vi "MB Embedded Modbus Demo Box Example.vi"() -> ()   [LabVIEW 2011]
uses:
  MB Serial Master Query Read Coils (poly).vi
  MB Serial Master Query Write Multiple Coils (poly).vi
  MB Serial Master Query Read Holding Registers (poly).vi
  MB Serial Master Query Write Multiple Registers (poly).vi
panel:
  in  "Stop":bool
  in  "COM Port":refnum<visa-resource-name>
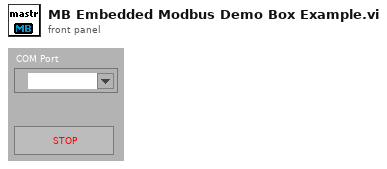
[diagram p1: front panel]
types:
  T1 = cluster{"Mode":enum16{"RTU", "ASCII"}, "Slave Address":u8}
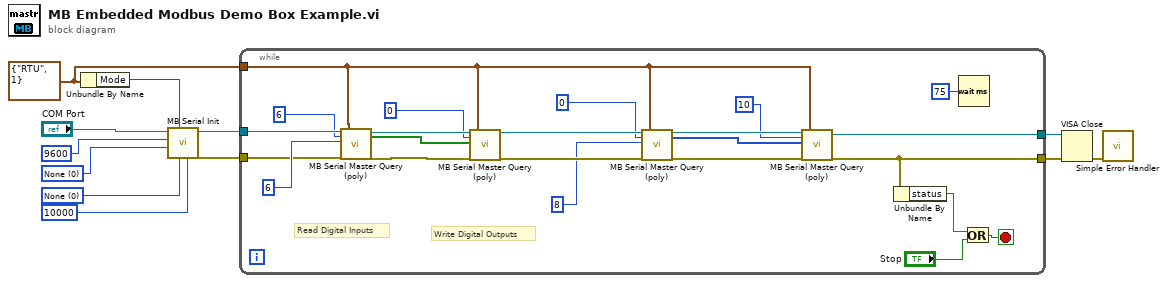
[diagram p0: block diagram]
diagram:
  w7 = u16 0 items=["None", "XON/XOFF", "RTS/CTS", "XON/XOFF & RTS/CTS", "DTR/DSR", "XON/XOFF & DTR/DSR"] ("Flow Control")
  w8 = u16 0 items=["None", "Odd", "Even", "Mark", "Space"] ("Parity")
  w4 = T1 {"Mode"=enum."RTU", "Slave Address"=1} ("Serial Parameters")
  n1 = Unbundle By Name(w4) -> ("Mode"=w10:enum16{"RTU", "ASCII"})
  n2 = call "MB Serial Init.vi"("Timeout"=u32 10000, "Flow Control"=w7, "Mode"=w10, "Parity"=w8, "Baud Rate"=u32 9600, "VISA resource name"="COM Port") -> ("error out"=w5:errorcluster, "VISA resource name out"=w11:refnum<visa-resource-name>)  [unwired: 1 in, 3 out]
  n3 = while {
    tunnel: w11 -> [w35]
    tunnel: w5 -> [w32]
    tunnel: w4 -> [w19]
    tunnel: [w15] -> w3
    tunnel: [w14] -> w2
    stop <- w18 stop-if-true
    # "Write Digital Outputs"
    # "Read Digital Inputs"
    n4 = call-poly "MB Serial Master Query (poly).vi"("VISA resource name"=w35, "Starting Address"=u16 6, "Quantity"=u16 6, "error in"=w32, "Serial Parameters"=w19) -> ("VISA resource name out"=w31:refnum<visa-resource-name>, "Coils"=w28:bool[], "error out"=w30:errorcluster)  [unwired: 1 in, 11 out]
    n5 = call-poly "MB Serial Master Query (poly).vi"("VISA resource name"=w31, "Starting Address"=u16 0, "Coils"=w28, "error in"=w30, "Serial Parameters"=w19) -> ("VISA resource name out"=w27:refnum<visa-resource-name>, "error out"=w26:errorcluster)  [unwired: 2 in, 11 out]
    n6 = call-poly "MB Serial Master Query (poly).vi"("VISA resource name"=w27, "Starting Address"=u16 0, "Quantity"=u16 8, "error in"=w26, "Serial Parameters"=w19) -> ("VISA resource name out"=w23:refnum<visa-resource-name>, "Holding Registers"=w20:u16[], "error out"=w22:errorcluster)  [unwired: 1 in, 11 out]
    n7 = call-poly "MB Serial Master Query (poly).vi"("VISA resource name"=w23, "Starting Address"=u16 10, "Registers"=w20, "error in"=w22, "Serial Parameters"=w19) -> ("VISA resource name out"=w14:refnum<visa-resource-name>, "error out"=w15:errorcluster)  [unwired: 2 in, 11 out]
    n8 = Unbundle By Name(w15) -> ("status"=w16:bool)
    n9 = Wait (ms)(milliseconds to wait=u32 75) -> ()  [unwired: 1 out]
    n10 = Or(x=w16, y="Stop") -> (x .or. y?=w18:bool)
  }
  n11 = VISA Close(VISA resource name=w2, error in (no error)=w3) -> (error out=w1:errorcluster)
  n12 = call <vilib>:"Simple Error Handler.vi"("error in (no error)"=w1) -> ()  [unwired: 1 in, 8 out]
